vi "h5_config_flatten_v2.vi"(8 "error in (no error)":errorcluster, 10 "scan_config":T1={"v0 name"="radiant (nm)", "v0 num"=808, "v1 name"="none", "v1 num"=808, "scan_values"=[], "num rows"=808, "measurement"=0, "v0_config"={"hardware"=enum."radiant (nm)", "options"="", "repeats"=4, "loops"=1, "VISA"="COM9", "override_VISA"=TRUE}, "v1_config"={"hardware"=enum."radiant (nm)", "options"="", "repeats"=4, "loops"=1, "VISA"="COM9", "override_VISA"=TRUE}, "scope_config"={"VISA"="lecroy", "channels"=[enum."Channel 1"], "timeout (ms)"=100000, "max_points"=2500, "averages"=50, "noise filter"=enum."None"}} {"scope_config"."averages" min=1; "scope_config"."max_points" items=["50"=50, "100"=100, "250"=250, "500"=500, "1000"=1000, "2500"=2500, "5K"=5000, "10K"=10000, "25K"=25000, "50K"=50000, "100K"=100000, "250K"=250000, "500K"=500000, "1M"=1000000, "2M"=2000000, "2.5M"=2500000, "5M"=5000000, "10M"=10000000, "25M"=25000000, "50M"=50000000, "100M"=100000000]; "v1_config"."loops" min=1; "v1_config"."repeats" min=1; "v0_config"."loops" min=1; "v0_config"."repeats" min=1}) -> (0 "error out":errorcluster, 1 "Values out":variant[](array[variant]), 2 "Names out":string[](array[string]))   [LabVIEW 2017, in "tools.lvlib"]
uses:
  tools.lvlib
  core/scan_config.ctl
  core/var_config.ctl
  ctrl/var_list.ctl
  hardware/lecroy/scope_config.ctl
  <vilib>/Utility/VariantDataType/GetClusterInfo.vi
  <vilib>/Utility/VariantDataType/GetTypeInfo.vi
  <vilib>/UPVI/lvhdf5/attribute.llb/Cluster to Attribute Array.xnode
  <vilib>/Utility/VariantDataType/VariantType.lvlib
  hardware/lecroy/lecroy.lvlib
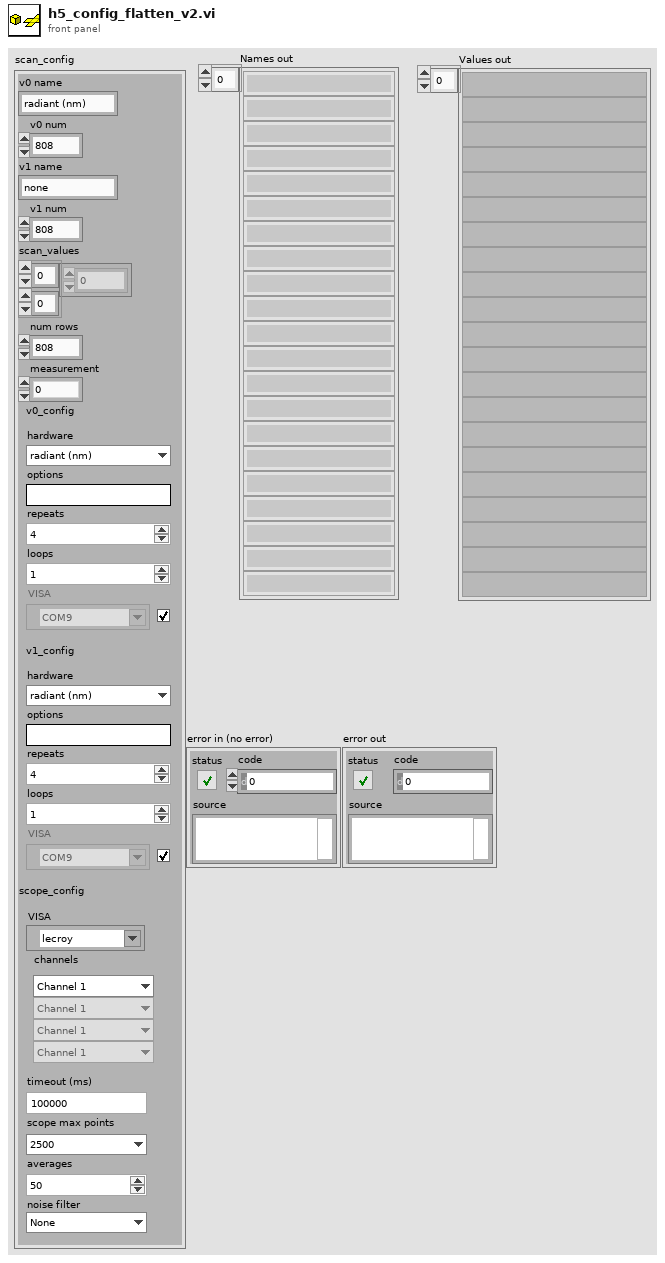
[diagram p1: front panel]
types:
  T1 = typedef "tools.lvlib/scan_config.ctl" = cluster{"v0 name":string, "v0 num":i32, "v1 name":string, "v1 num":i32, "scan_values":dbl[][], "num rows":i32, "measurement":i32, "v0_config":T2, "v1_config":T2, "scope_config":T4}
  T2 = typedef "tools.lvlib/var_config.ctl" = cluster{"hardware":T3, "options":string, "repeats":i32, "loops":i32, "VISA":refnum<visa-resource-name>, "override_VISA":bool}
  T3 = typedef "var_list.ctl" = enum16{"none", "AO voltage (V)", "delay (s)", "generic", "microwaves (GHz)", "radiant (nm)", "radiant thg (nm)", "sirah (nm)", "sirah_shg (nm)", "tenma voltage (V)", "wait (s)", "wf_freq (Hz)", "wf_amp (V)", "wf_amp_multi (V)", "wf_offset (V)", "wf_low_level (V)", "wf_high_level (V)", "wf_period (s)", "wf_pulse_width (s)", "wf_sample_rate (Sa/s)", "wf_multi_amp", "wf_multi_freq", "wf_arb_4chan", "WS7 setpoint (nm)"}
  T4 = typedef "lecroy.lvlib/scope_config.ctl" = cluster{"VISA":refnum<visa-resource-name>, "channels":enum16{"Channel 1", "Channel 2", "Channel 3", "Channel 4"}[], "timeout (ms)":u32, "max_points":i32, "averages":i32, "noise filter":enum16{"None", "+0.5 bit", "+1 bit", "+1.5 bits", "+2 bits", "+2.5 bits", "+3 bits"}}
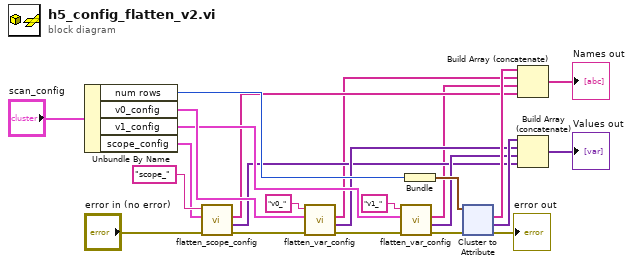
[diagram p0: block diagram]
diagram:
  n1 = Unbundle By Name("scan_config") -> ("num rows"=w23:i32, "v0_config"=w18:T2, "v1_config"=w15:T2, "scope_config"=w13:T4)
  n2 = call "flatten_scope_config.vi"("error in (no error)"="error in (no error)", "scope_config"=w13, "name"="scope_") -> ("error out"=w11:errorcluster, "values"=w7:variant[], "names"=w6:string[])  [unwired: 6 in]
  n3 = call "flatten_var_config.vi"("error in (no error)"=w11, "var_config"=w18, "name"="v0_") -> ("error out"=w10:errorcluster, "values"=w9:variant[], "names"=w4:string[])  [unwired: 6 in]
  n4 = call "flatten_var_config.vi"("error in (no error)"=w10, "var_config"=w15, "name"="v1_") -> ("error out"=w2:errorcluster, "values"=w8:variant[], "names"=w5:string[])  [unwired: 6 in]
  n5 = Bundle("num rows"=w23) -> (w22:cluster{"num rows":i32})  [unwired: 1 in]
  n6 = xnode "Cluster to Attribute"("error in (no error)"=w2, "Cluster"=w22) -> ("Names out"=w21:string[], "Values out"=w20:variant[], "error out"=→"error out":errorcluster)  [unwired: 4 in]
  n7 = Build Array (concatenate)(w21, w4, w5, w6) -> (→"Names out":string[])
  n8 = Build Array (concatenate)(w20, w9, w8, w7) -> (→"Values out":variant[])
